vi "SIG_Test.vi"() -> ()   [LabVIEW 2014]
panel:
  out "size(s)":i32
  out "SIG valid?":bool
  out "original bit numbers":u32
  out "encoded bit numbers":u32
  out "Symbol numbers":i32
  out "Modulation parameter 2":T1
  in  "Data bit length":i32
  in  "Modulation parameter":T1
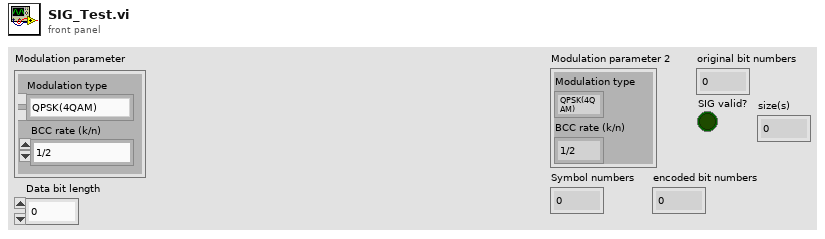
[diagram p1: front panel]
types:
  T1 = cluster{"Modulation type":enum16{"QPSK(4QAM)", "64QAM", "16QAM", "BPSK"}, "BCC rate (k/n)":enum16{"1/2", "2/3", "3/4"}}
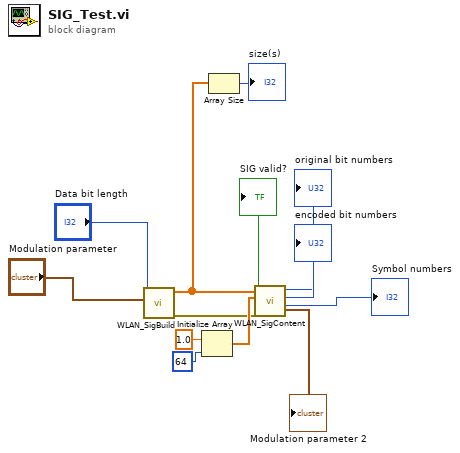
[diagram p0: block diagram]
diagram:
  n1 = call "WLAN_SigBuild.vi"("Data bit length"="Data bit length", "Modulation parameter"="Modulation parameter") -> ("symbols"=w2:cdb[], "error out"=w8:errorcluster)  [unwired: 7 in]
  n2 = Initialize Array(1.0 ("element"), 64 ("dimension size")) -> (w13:dbl[])
  n3 = Array Size(array=w2) -> (size(s)=→"size(s)":i32)
  n4 = call "WLAN_SigContent.vi"("error in (no error)"=w8, "Frequency channel estimation"=w13, "SIG"=w2) -> ("Symbol numbers"=→"Symbol numbers":i32, "encoded bit numbers"=→"encoded bit numbers":u32, "original bit numbers"=→"original bit numbers":u32, "Modulation parameter"=→"Modulation parameter 2":T1, "SIG valid?"=→"SIG valid?":bool)  [unwired: 3 in, 1 out]
